vi "FeedbackDecode_KalmanEMG2Str.vi"(1 "KalmanEMG":T1) -> (0 "KalmanEMGStr":string)   [LabVIEW 2020]
panel:
  # "1"
  # "2"
  # "3"
  # "4"
  # "5"
  # "6"
  # "7"
  # "8"
  # "1"
  # "2"
  # "3"
  # "4"
  # "1-2"
  # "1-3"
  # "1-4"
  # "2-3"
  # "2-4"
  # "3-4"
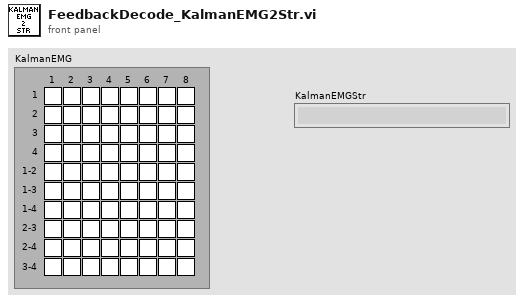
[diagram p1: front panel]
types:
  T1 = cluster{"Boolean 92":bool, "Boolean 82":bool, "Boolean 72":bool, "Boolean 62":bool, "Boolean 52":bool, "Boolean 42":bool, "Boolean 32":bool, "Boolean 22":bool, "Boolean 12":bool, "Boolean 2":bool, "Boolean 93":bool, "Boolean 83":bool, "Boolean 73":bool, "Boolean 63":bool, "Boolean 53":bool, "Boolean 43":bool, "Boolean 33":bool, "Boolean 23":bool, "Boolean 13":bool, "Boolean 3":bool, "Boolean 94":bool, "Boolean 84":bool, "Boolean 74":bool, "Boolean 64":bool, "Boolean 54":bool, "Boolean 44":bool, "Boolean 34":bool, "Boolean 24":bool, "Boolean 14":bool, "Boolean 4":bool, "Boolean 95":bool, "Boolean 85":bool, "Boolean 75":bool, "Boolean 65":bool, "Boolean 55":bool, "Boolean 45":bool, "Boolean 35":bool, "Boolean 25":bool, "Boolean 15":bool, "Boolean 5":bool, "Boolean 96":bool, "Boolean 86":bool, "Boolean 76":bool, "Boolean 66":bool, "Boolean 56":bool, "Boolean 46":bool, "Boolean 36":bool, "Boolean 26":bool, "Boolean 16":bool, "Boolean 6":bool, "Boolean 97":bool, "Boolean 87":bool, "Boolean 77":bool, "Boolean 67":bool, "Boolean 57":bool, "Boolean 47":bool, "Boolean 37":bool, "Boolean 27":bool, "Boolean 17":bool, "Boolean 7":bool, "Boolean 98":bool, "Boolean 88":bool, "Boolean 78":bool, "Boolean 68":bool, "Boolean 58":bool, "Boolean 48":bool, "Boolean 38":bool, "Boolean 28":bool, "Boolean 18":bool, "Boolean 8":bool, "Boolean 99":bool, "Boolean 89":bool, "Boolean 79":bool, "Boolean 69":bool, "Boolean 59":bool, "Boolean 49":bool, "Boolean 39":bool, "Boolean 29":bool, "Boolean 19":bool, "Boolean 9":bool}
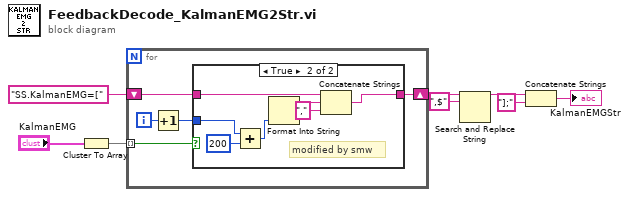
[diagram p0: block diagram]
diagram:
  n1 = Cluster To Array(cluster="KalmanEMG") -> (array=w8:bool[])
  n2 = for {
    shift-right: [w12] -> w3
    shift-left: "SS.KalmanEMG=[" -> [w13]
    tunnel: w8 -> [w10] mode=indexing
    i -> [w11]
    n3 = Increment(x=w11) -> (x+1=w9:i32)
    n4 = case shown="True" w10 {
      tunnel: w13 -> [w14 w21]
      tunnel: [w14 w20] -> w12
      tunnel: w9 -> [_ w17]
      frame False {
      }
      frame True {
        # "modified by smw"
        n5 = Add(x=w17, y=200) -> (x+y=w15:i32)
        n6 = Format Into String(w15) -> (resulting string=w19:string)  [unwired: 3 in, 1 out]
        n7 = Concatenate Strings(w21, w19, "," ("string")) -> (w20:string)
      }
    }
  }
  n8 = Search and Replace String(input string=w3, search string=",$") -> (result string=w5:string)  [unwired: 6 in, 3 out]
  n9 = Concatenate Strings(w5, "];" ("string")) -> (→"KalmanEMGStr":string)
